vi "GetGrabberPositions.vi"(0 "reference":refnum<class "RectangularNode.lvclass">, 5 "error in (no error)":errorcluster) -> (14 "reference out":refnum<class "RectangularNode.lvclass">, 15 "GrabberPositions":T2[](array[typedef]) {"y" format="%.2f"; "x" format="%.2f"}, 16 "HotSpots":T1[](array[typedef]) {"HotSpot"."y" format="%.2f"; "HotSpot"."x" format="%.2f"}, 19 "error out":errorcluster)   [LabVIEW 2020, in "RectangularNode.lvclass"]
doc: "public Rectangle2D getBounds(Graphics2D g2)"
uses:
  <resource>/Framework/Providers/Open_GDS/UML/RectangularNode_class/RectangularNode.lvclass
  <resource>/Framework/Providers/Open_GDS/UML/General/Point/Point Point2D.ctl
  <resource>/Framework/Providers/Open_GDS/UML/UMLEditor/UMLEditor_HotSpotData.ctl
  <resource>/Framework/Providers/Open_GDS/UML/AbstractNode_class/AbstractNode.lvclass
  <resource>/Framework/Providers/Open_GDS/UML/UMLEditor/UMLEditor_HotSpotType.ctl
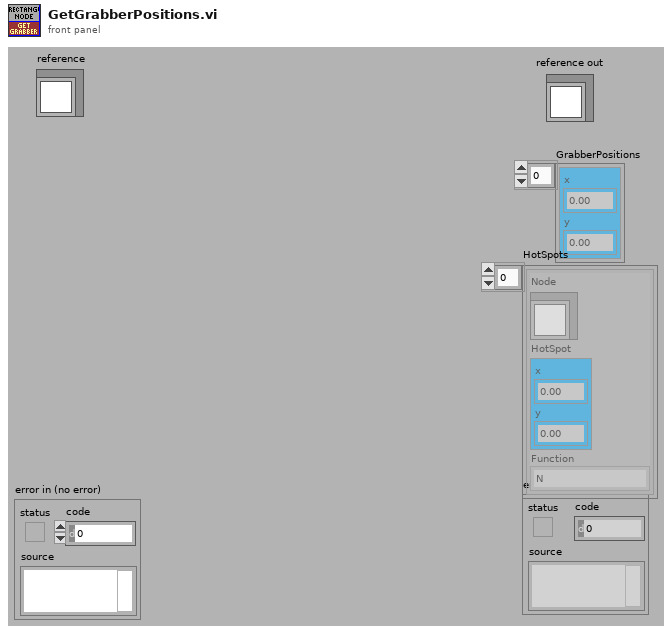
[diagram p1: front panel]
types:
  T1 = typedef "UMLEditor_HotSpotData.ctl" = cluster{"Node":refnum<class "AbstractNode.lvclass">, "HotSpot":T2, "Function":T3}
  T2 = typedef "Point Point2D.ctl" = cluster{"x":dbl, "y":dbl}
  T3 = typedef "UMLEditor_HotSpotType.ctl" = enum16{"N", "NE", "E", "SE", "S", "SW", "W", "NW", "Expand", "Collaps"}
  T4 = typedef "Rectangle Rectangle2D.ctl" = cluster{"x":dbl, "y":dbl, "width":dbl, "height":dbl}
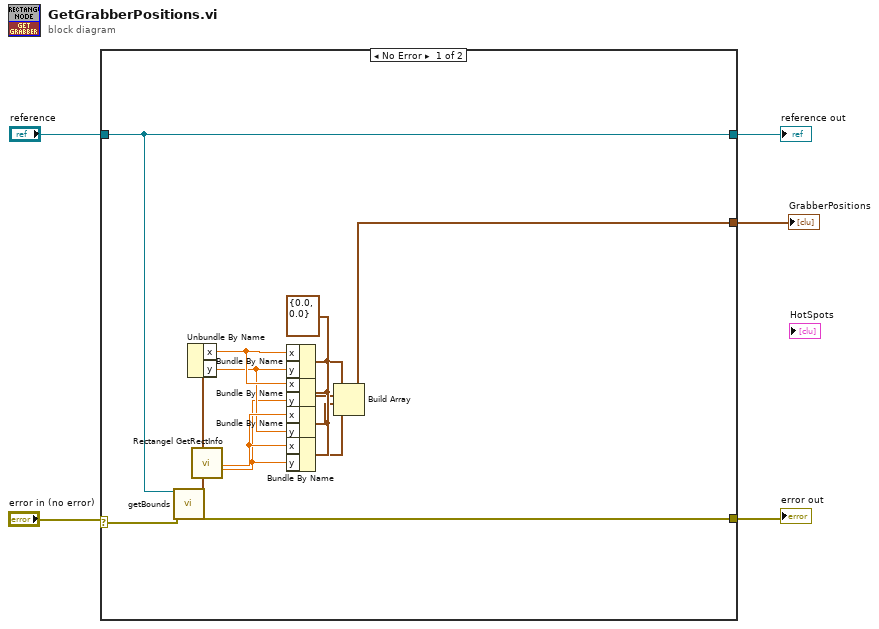
[diagram p0: block diagram]
diagram:
  n1 = case shown="No Error" "error in (no error)" {
    selector: "error in (no error)" -> [w8 w20]
    tunnel: "reference" -> [w6 w21]
    tunnel: [w9 w20] -> w4
    tunnel: [w6 w21] -> w3
    tunnel: [w7 _] -> w1
    frame No Error {
      w19 = T2 {"x"=0.0, "y"=0.0} ("point2D")
      n2 = call-dynamic "getBounds.vi"("reference"=w6, "error in (no error)"=w8) -> ("bounds"=w18:T4, "error out"=w9:errorcluster)  [unwired: 15 in, 1 out]
      n3 = Unbundle By Name(w18) -> ("x"=w17:dbl, "y"=w15:dbl)
      n4 = call <resource>:"Rectangel GetRectInfo.vi"("bounds"=w18) -> ("maxX"=w16:dbl, "maxY"=w14:dbl)  [unwired: 1 in, 16 out]
      n5 = Bundle By Name(cluster=w19, "x"=w17, "y"=w15) -> (w13:T2)
      n6 = Bundle By Name(cluster=w19, "x"=w17, "y"=w14) -> (w12:T2)
      n7 = Bundle By Name(cluster=w19, "x"=w16, "y"=w15) -> (w11:T2)
      n8 = Bundle By Name(cluster=w19, "x"=w16, "y"=w14) -> (w10:T2)
      n9 = Build Array(w13, w12, w11, w10) -> (w7:T2[])
    }
    frame Error {
    }
  }
  "reference out" <- w3
  "error out" <- w4
  "GrabberPositions" <- w1
